vi "IR wall.vi"(2 "Banchmark in":T2={"DC estimate (V)2"=1.2526850823671394, "DC estimate (V)1"=2.565470433392377}, 3 "IR in":T1) -> (0 "result":dbl[](array[numeric]), 1 "x > y?":bool)   [LabVIEW 2019]
uses:
  alignment benchmark.ctl
  distance measure/IR/IR out.ctl
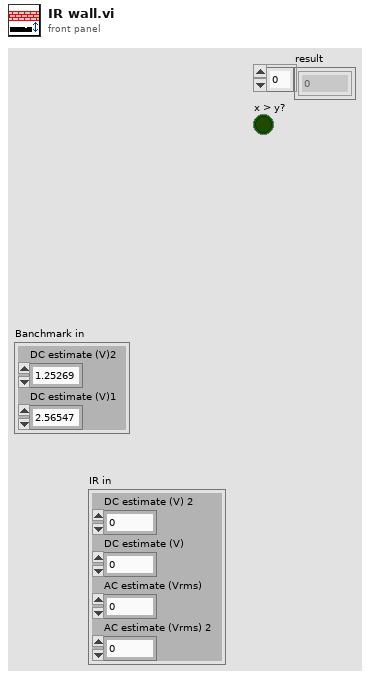
[diagram p1: front panel]
types:
  T1 = typedef "IR out.ctl" = cluster{"DC estimate (V) 2":dbl, "DC estimate (V)":dbl, "AC estimate (Vrms)":dbl, "AC estimate (Vrms) 2":dbl}
  T2 = typedef "alignment benchmark.ctl" = cluster{"DC estimate (V)2":dbl, "DC estimate (V)1":dbl}
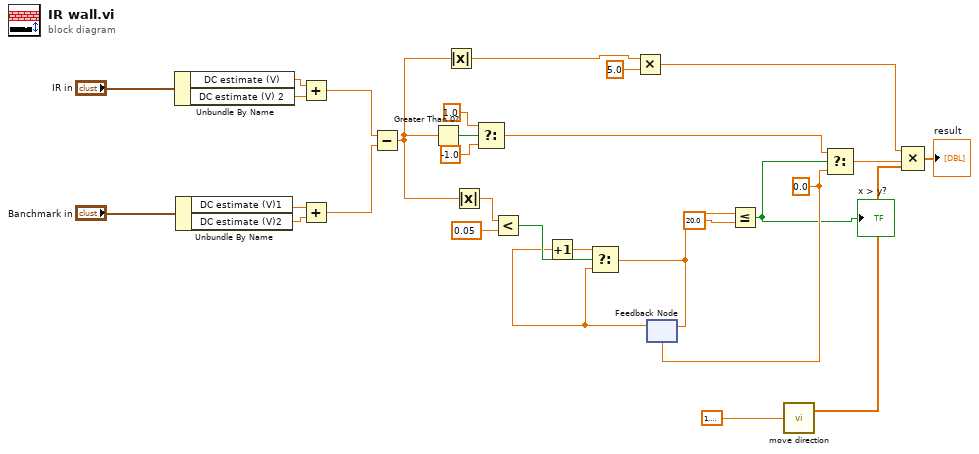
[diagram p0: block diagram]
diagram:
  w8 = 0.0 ("f")
  n1 = Unbundle By Name("IR in") -> ("DC estimate (V)"=w24:dbl, "DC estimate (V) 2"=w25:dbl)
  n2 = Unbundle By Name("Banchmark in") -> ("DC estimate (V)1"=w27:dbl, "DC estimate (V)2"=w26:dbl)
  n3 = Add(x=w24, y=w25) -> (x+y=w23:dbl)
  n4 = Add(x=w27, y=w26) -> (x+y=w22:dbl)
  n5 = Subtract(x=w23, y=w22) -> (x-y=w9:dbl)
  n6 = Greater Than 0?(x=w9) -> (x > 0?=w12:bool)
  n7 = Absolute Value(x=w9) -> (abs(x)=w10:dbl)
  n8 = Absolute Value(x=w9) -> (abs(x)=w21:dbl)
  n9 = Select(t=1.0 ("f"), s=w12, f=-1.0) -> (s? t:f=w7:dbl)
  n10 = Less?(x=w21, y=0.05) -> (x < y?=w19:bool)
  n11 = Multiply(x=w10, y=5.0) -> (x*y=w3:dbl)
  n12 = feedback #1(w8) -> (w17:dbl)
  n13 = Increment(x=w17) -> (x+1=w18:dbl)
  n14 = Select(t=w18, s=w19, f=w17) -> (s? t:f=w16:dbl)
  n15 = feedback-in #1(w16) -> ()
  n16 = Less Or Equal?(x=w16, y=20.0) -> (x <= y?=w1:bool)
  "x > y?" <- w1
  n17 = call "move direction.vi"("theta"=1.5707963267948966) -> ("out array"=w6:dbl[])  [unwired: 1 out]
  n18 = Select(t=w7, s=w1, f=w8) -> (s? t:f=w4:dbl)
  n19 = Compound Arithmetic op=MULTIPLY(w3, w4, w6) -> (→"result":dbl[])
